vi "Wall-E.vi"() -> ()   [LabVIEW 2014]
doc: "Tank Drive Example\n\nThis example shows how to implement tank drive and uses two joysticks for input.\n\nThis example expects a USB cable connected from your development PC to the Type B USB Jack (next to the power input) on the roboRIO.\n\nThis example requires the Driver Station to be running with Teleoperated Enabled."
uses:
  <vilib>/Rock Robotics/SystemInterfaces/DIO/FPGA_DIOPWMChannel.ctl
  <vilib>/Rock Robotics/WPI/Joystick/WPI_JoystickDeviceEnum.ctl
  <vilib>/Rock Robotics/WPI/Solenoid/WPI_SolenoidChannel.ctl
  <vilib>/Rock Robotics/WPI/Solenoid/WPI_SolenoidValue.ctl
  <vilib>/Rock Robotics/WPI/MotorControl/WPI_MotorControlOpen Talon.vi
  <vilib>/Rock Robotics/WPI/Solenoid/WPI_SolenoidOpenDouble.vi
  <vilib>/Rock Robotics/WPI/RobotDrive/WPI_RobotDriveOpen4MotorWithTalon.vi
  <vilib>/Rock Robotics/WPI/Solenoid/WPI_SolenoidSetEnum.vi
panel:
  in  "stop":bool
  # "Set these inputs before running."
  # "This example requires the Driver Station to be running with Teleoperated Enabled."
  # "PWM cables"
  # "This shows wiring for Talon speed controllers.  The wiring is similar for Victor and Jaguar controllers.  If you change the controller type, you must also select the appropriate instance of the Motor Open VI on the diagram."
  # "Power\nTerminals"
  # "Motor\nTerminals"
  # "+"
  # "+"
  # "M"
  # "B"
  # "Power\nTerminals"
  # "Motor\nTerminals"
  # "+"
  # "+"
  # "M"
  # "B"
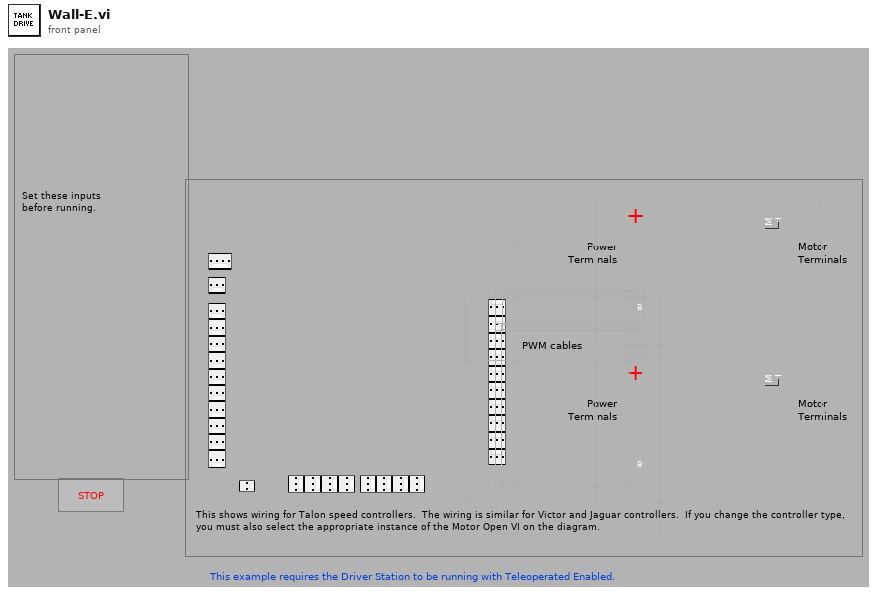
[diagram p1: front panel]
types:
  T1 = typedef "WPI_SolenoidChannel.ctl" = enum8{"Solenoid 0", "Solenoid 1", "Solenoid 2", "Solenoid 3", "Solenoid 4", "Solenoid 5", "Solenoid 6", "Solenoid 7", "Invalid"}
  T2 = typedef "WPI_JoystickDeviceEnum.ctl" = enum16{"USB 0", "USB 1", "USB 2", "USB 3", "USB 4", "USB 5"}
  T3 = typedef "FPGA_DIOPWMChannel.ctl" = enum8{"PWM 0", "PWM 1", "PWM 2", "PWM 3", "PWM 4", "PWM 5", "PWM 6", "PWM 7", "PWM 8", "PWM 9", "PWM MXP 0", "PWM MXP 1", "PWM MXP 2", "PWM MXP 3", "PWM MXP 4", "PWM MXP 5", "PWM MXP 6", "PWM MXP 7", "PWM MXP 8", "PWM MXP 9", "Invalid"}
  T4 = typedef "WPI_JoystickDevRef.ctl" = cluster{"Device":T2}
  T5 = typedef "WPI_SolenoidDevRef.ctl" = cluster{"DevStatus":errorcluster, "Pneumatics Control Module":u8, "Forward Solenoid Channel":T1, "Reverse Solenoid Channel":T1}
  T6 = typedef "WPI_MotorControlDeviceRef.ctl" = cluster{"DeviceStatus":errorcluster, "Type":T7, "PWM":cluster{"Controller":T8, "PWM Channel":T3, "DeadBand":T9}, "CAN":cluster{"Device Number":u8, "Control Mode":T10, "Semaphore":T11, "Max Vout":dbl, "TalonSRX Control Mode":T12}, "Invert":bool, "TransformRef":T13, "InvTransformRef":T13}
  T7 = typedef "WPI_MotorControlType.ctl" = enum16{"PWM", "CAN", "CANTalonSRX"}
  T8 = typedef "FPGA_TypedefDigitalModule.ctl" = enum16{"Controller 1"}
  T9 = typedef "WPI_PWMDeadband.ctl" = cluster{"Name":string, "maxPositivePwm":i32, "minPositivePwm":i32, "centerPwm":i32, "maxNegativePwm":i32, "minNegativePwm":i32, "angularRange":u16}
  T10 = typedef "WPI_CANJaguar_ControlMode.ctl" = enum8{"Percent VBus", "Current", "Speed", "Position", "Voltage"}
  T11 = typedef "Semaphore RefNum" = refnum<k1>
  T12 = typedef "WPI_CANTalonSRX_APIControlMode.ctl" = enum8{"Percent VBus", "Speed", "Position", "Slave", "Unchanged / Invalid"}
  T13 = typedef "WPI_PWMTransform_ConPane.ctl" = refnum<vi>
  T14 = typedef "WPI_RobotDriveDevRef.ctl" = cluster{"DevStatus":errorcluster, "Motors[]":T6[], "Square Inputs":bool, "Max Output":dbl}
  T15 = typedef "WPI_SolenoidValue.ctl" = enum16{"Off", "On", "Forward", "Reverse"}
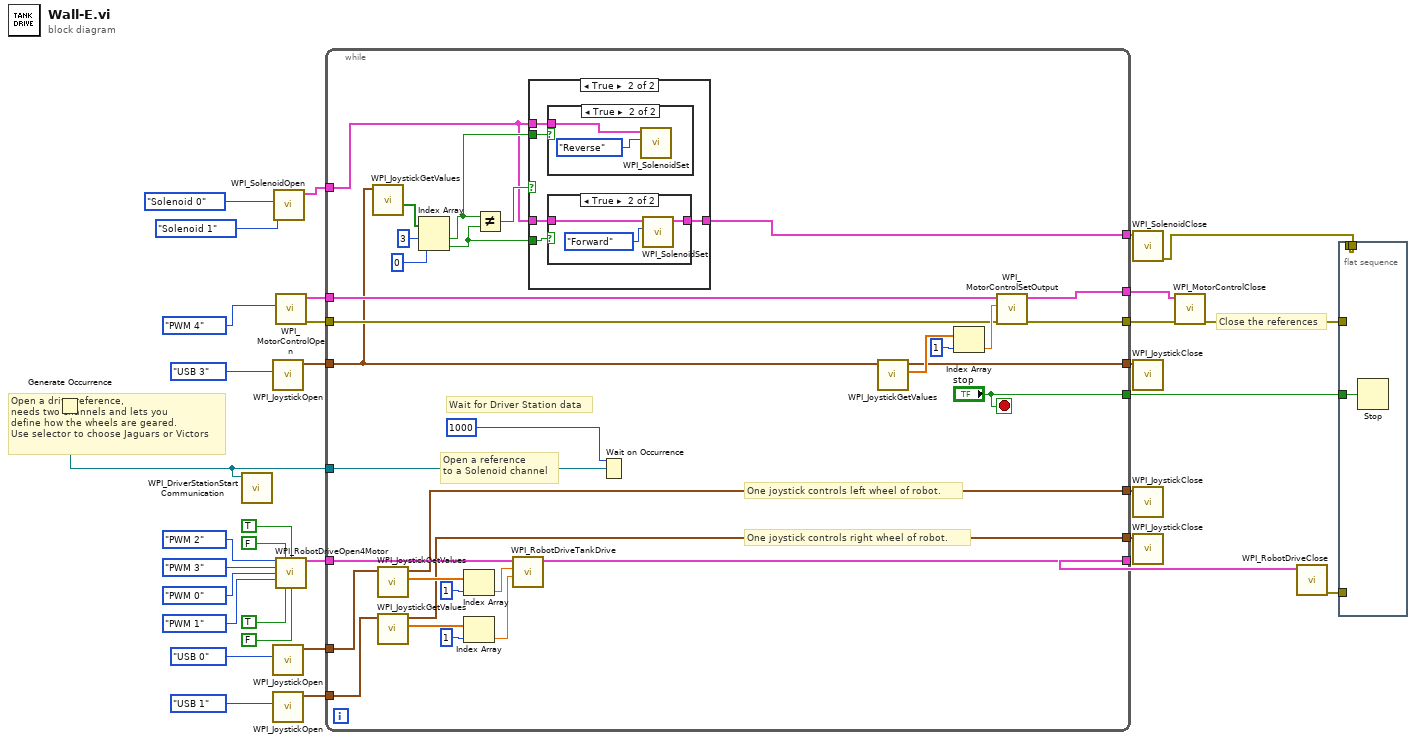
[diagram p0: block diagram]
diagram:
  # "Close the references"
  # "Open a drive reference,\nneeds two channels and lets you\ndefine how the wheels are geared.\nUse selector to choose Jaguars or Victors"
  n1 = Generate Occurrence() -> (w32:refnum<k4>)
  n2 = call <vilib>:"WPI_DriverStationStart Communication.vi"("occurrence"=w32) -> ()  [unwired: 1 in, 10 out]
  n3 = call <vilib>:"WPI_JoystickOpen.vi"("JoystickDevice"=WPI_JoystickDeviceEnum."USB 3") -> ("JoystickDevRef"=w12:T4)  [unwired: 10 out]
  n4 = call <vilib>:"WPI_JoystickOpen.vi"("JoystickDevice"=WPI_JoystickDeviceEnum."USB 0" ("LeftStick")) -> ("JoystickDevRef"=w28:T4)  [unwired: 10 out]
  n5 = call <vilib>:"WPI_JoystickOpen.vi"("JoystickDevice"=WPI_JoystickDeviceEnum."USB 1" ("RightStick")) -> ("JoystickDevRef"=w29:T4)  [unwired: 10 out]
  n6 = call-poly <vilib>:"WPI_SolenoidOpen.vi"("Reverse Solenoid Channel"=WPI_SolenoidChannel."Solenoid 1", "Forward Solenoid Channel"=WPI_SolenoidChannel."Solenoid 0" ("Solenoid Channel")) -> ("SolenoidDevRef"=w7:T5)  [unwired: 8 in, 1 out]
  n7 = call-poly <vilib>:"WPI_MotorControlOpen.vi"("PWM Channel"=FPGA_DIOPWMChannel."PWM 4" ("Right Motor")) -> ("error out"=w1:errorcluster, "MotorControlDeviceRef"=w10:T6)  [unwired: 9 in]
  n8 = call-poly <vilib>:"WPI_RobotDriveOpen4Motor.vi"("Rear Left Motor"=FPGA_DIOPWMChannel."PWM 2" ("Left Motor (PWM channel)"), "Rear Left Motor Inverted"=FALSE, "Rear Right Motor Inverted"=TRUE, "Rear Right Motor"=FPGA_DIOPWMChannel."PWM 3" ("Right Motor (PWM channel)"), "Front Left Motor"=FPGA_DIOPWMChannel."PWM 0", "Front Right Motor"=FPGA_DIOPWMChannel."PWM 1", "Front Left Motor Inverted"=TRUE, "Front Right Motor Inverted"=FALSE) -> ("RobotDriveDevRef"=w21:T14)  [unwired: 6 in, 1 out]
  n9 = while {
    tunnel: w21 -> [w60]
    tunnel: [w61] -> w33
    tunnel: w32 -> [w65]
    tunnel: ["stop"] -> w25
    tunnel: w29 -> [w63]
    tunnel: w28 -> [w62]
    tunnel: [w58] -> w27
    tunnel: [w57] -> w26
    tunnel: [w35] -> w15
    tunnel: [w49] -> w13
    tunnel: w12 -> [w39]
    tunnel: w10 -> [w42]
    tunnel: [w48] -> w3
    tunnel: w7 -> [w34]
    tunnel: [w41] -> w2
    tunnel: w1 -> [w40]
    stop <- "stop" stop-if-true
    # "Open a reference \nto a Solenoid channel"
    # "Wait for Driver Station data"
    # "One joystick controls right wheel of robot."
    # "One joystick controls left wheel of robot."
    n10 = call <vilib>:"WPI_JoystickGetValues.vi"("JoystickDevRef"=w39) -> ("Buttons"=w44:bool[])  [unwired: 6 in, 4 out]
    n11 = call <vilib>:"WPI_JoystickGetValues.vi"("JoystickDevRef"=w62) -> ("Axes"=w59:dbl[], "JoystickDevRef"=w58:T4)  [unwired: 6 in, 3 out]
    n12 = call <vilib>:"WPI_JoystickGetValues.vi"("JoystickDevRef"=w63) -> ("Axes"=w54:dbl[], "JoystickDevRef"=w57:T4)  [unwired: 6 in, 3 out]
    n13 = Index Array(array=w44, index #1=3 ("index"), index #2=0 ("index")) -> (element #1=w37:bool, element #2=w36:bool)
    n14 = Index Array(array=w59, index=1) -> (element=w53:dbl)
    n15 = Index Array(array=w54, index=1) -> (element=w52:dbl)
    n16 = Not Equal?(x=w37, y=w36) -> (x != y?=w38:bool)
    n17 = call <vilib>:"WPI_RobotDriveTankDrive.vi"("Right axis value"=w52, "Left axis value"=w53, "RobotDriveDevRef"=w60) -> ("RobotDriveDevRef"=w61:T14)  [unwired: 6 in, 2 out]
    n18 = case shown="True" w38 {
      tunnel: w37 -> [_ w71]
      tunnel: w36 -> [_ w70]
      tunnel: [w66 w69] -> w35
      tunnel: w34 -> [_ w68]
      tunnel: w34 -> [w66 w67]
      frame False {
      }
      frame True {
        n19 = case shown="True" w71 {
          tunnel: w68 -> [_ w77]
          frame False {
          }
          frame True {
            n20 = call-poly <vilib>:"WPI_SolenoidSet.vi"("Value"=WPI_SolenoidValue."Reverse", "SolenoidDevRef"=w77) -> ()  [unwired: 1 in, 9 out]
          }
        }
        n21 = case shown="True" w70 {
          tunnel: [w72 w75] -> w69
          tunnel: w67 -> [w72 w74]
          frame False {
          }
          frame True {
            n22 = call-poly <vilib>:"WPI_SolenoidSet.vi"("Value"=WPI_SolenoidValue."Forward", "SolenoidDevRef"=w74) -> ("SolenoidDevRef"=w75:T5)  [unwired: 1 in, 8 out]
          }
        }
      }
    }
    n23 = Wait on Occurrence(2:w65, 3:1000 ("ms timeout (-1)")) -> ()  [unwired: 2 out]
    n24 = call <vilib>:"WPI_JoystickGetValues.vi"("JoystickDevRef"=w39) -> ("Axes"=w50:dbl[], "JoystickDevRef"=w49:T4)  [unwired: 6 in, 3 out]
    n25 = Index Array(array=w50, index=1) -> (element=w46:dbl)
    n26 = call <vilib>:"WPI_MotorControlSetOutput.vi"("error in (no error)"=w40, "Output"=w46, "MotorControlDevRef"=w42) -> ("error out"=w41:errorcluster, "MotorControlDevRef"=w48:T6)  [unwired: 6 in, 1 out]
  }
  n27 = call <vilib>:"WPI_SolenoidClose.vi"("SolenoidDevRef"=w15) -> ("error out"=w6:errorcluster)  [unwired: 10 in]
  n28 = call <vilib>:"WPI_JoystickClose.vi"("JoystickDevRef"=w13) -> ()  [unwired: 11 in]
  n29 = call <vilib>:"WPI_JoystickClose.vi"("JoystickDevRef"=w27) -> ()  [unwired: 11 out]
  n30 = call <vilib>:"WPI_JoystickClose.vi"("JoystickDevRef"=w26) -> ()  [unwired: 11 out]
  n31 = call <vilib>:"WPI_MotorControlClose.vi"("error in (no error)"=w2, "MotorControlDevRef"=w3) -> ("error out"=w11:errorcluster)  [unwired: 9 in]
  n32 = call <vilib>:"WPI_RobotDriveClose.vi"("RobotDriveDevRef"=w33) -> ("error out"=w24:errorcluster)  [unwired: 10 in]
  n33 = flat-sequence {
    tunnel: w25 -> [w79]
    tunnel: w24 -> [_]
    tunnel: w11 -> [_]
    tunnel: [w78] -> _
    tunnel: w6 -> [w78]
    frame #0 {
      n34 = Stop(stop? (T)=w79) -> ()
    }
  }
